vi "Pulse Attribute, Calculate Relative Time.vi"(6 "error in":errorcluster, 8 "index":dbl=5000.5 min=3.0 format="%.3f", 9 "waveform":waveform(dbl)={"t0"=timestamp(3472747248.0780005 s since 1904-01-01), "dt"=2e-06, "Y"=[]}) -> (0 "error out":errorcluster, 2 "relative time (s)":dbl=nan min=3.0 format="%.6f", 3 "waveform dup":waveform(dbl)={"t0"=timestamp(0 s since 1904-01-01), "dt"=nan, "Y"=[]})   [LabVIEW 2010]
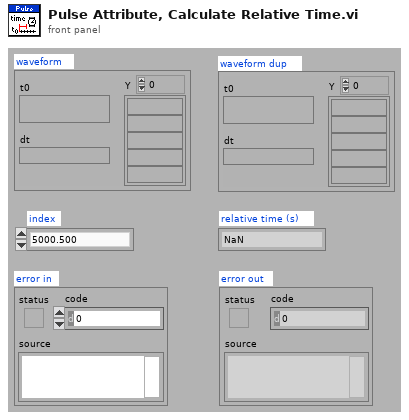
[diagram p1: front panel]
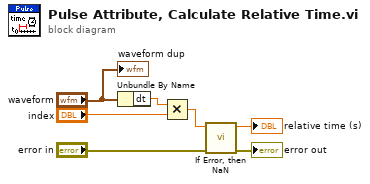
[diagram p0: block diagram]
diagram:
  n1 = Unbundle By Name("waveform") -> ("dt"=w5:dbl)
  n2 = Multiply(x=w5, y="index") -> (x*y=w2:dbl)
  n3 = call "If Error, then NaN.vi"("error in (T)"="error in", "value1"=w2) -> ("error out"=→"error out":errorcluster, "value out1"=→"relative time (s)":dbl)  [unwired: 4 in, 2 out]
  "waveform dup" <- "waveform"
